vi "Actor Core.vi"(8 "error in":errorcluster, 11 "Camera in":refnum<class "Camera.lvclass">) -> (0 "error out":errorcluster, 3 "Actor out":refnum<class "Actor.lvclass">)   [LabVIEW 2021, in "Camera.lvlib" / "Camera.lvclass"]
doc: "(<B>Filename</B>: Actor Framework.lvlib:Actor.lvclass:Actor Core.vi)\n\nReceives messages to the actor, reacts to them, and initiates any error handling that may shut the actor down.\n\nDescendant classes may override this VI to append parallel tasks for the actor to complete while it handles messages. Overrides use the Call Parent Method node."
uses:
  Camera.lvclass
  C:/Program Files (x86)/National Instruments/LabVIEW 2021/vi.lib/ActorFramework/Actor/Actor.lvclass
  <vilib>/ActorFramework/Actor/Actor.lvclass
  Cam task parameters.ctl
  Display Mode.ctl
  <vilib>/vision/Image Controls.llb/IMAQ Image.ctl
  Utilities/RWC_Actions.ctl
  Camera.lvclass/Camera.ctl
  <vilib>/ActorFramework/Actor/Actor.lvclass/Actor.ctl
  <vilib>/ActorFramework/Message Enqueuer/Message Enqueuer.lvclass/Message Enqueuer.ctl
  Main_Control/Main_Control/notifications.ctl
  Main_Control/Main_Control Messages/UI notifier Msg/UI notifier Msg.lvclass/UI notifier Msg.ctl
  Camera Messages/Cam save image Msg/Cam save image Msg.lvclass/Cam save image Msg.ctl
  <vilib>/ActorFramework/Message Enqueuer/Init from Existing Queue.vi
  <vilib>/ActorFramework/Message Enqueuer/Enqueue.vi
  Camera Messages/Cam change inner param Msg/Cam change inner param Msg.lvclass
  C:/Program Files (x86)/National Instruments/LabVIEW 2021/vi.lib/ActorFramework/Message/Message.lvclass
  Camera Messages/Cam stop task Msg/Cam stop task Msg.lvclass
  Main_Control/Main_Control Messages/UI notifier Msg/UI notifier Msg.lvclass
  Camera Messages/Cam save image Msg/Cam save image Msg.lvclass
  <vilib>/ActorFramework/Message Priority Queue/Priority Enqueue.vi
  <vilib>/ActorFramework/Message Enqueuer/Message Enqueuer.lvclass
  Main_Control/Main_Control/Main_Control.lvclass
panel:
  out "Waveform Graph":dbl[](graph)
  in  "stop":bool
  in  "Change inner param":bool
  in  "Frame Array":T1[](array[typedef])
  in  "Max":u16(slide) scale=0.0..65535.0
  in  "Min":u16(slide) scale=0.0..65535.0
  in  "phase display":i32
  in  "phase#":i32=1
  in  "Display Index":u32(slide) scale=0.0..10.0
  in  "Display Mode":T2
  out "Image":T1(plugin-control)
  in  "Cam task parameters":T3
  out "Current Frame":i32
  out "Exposure Index":i32
  in  "Auto Saving?":bool
  in  "Is Running?":bool
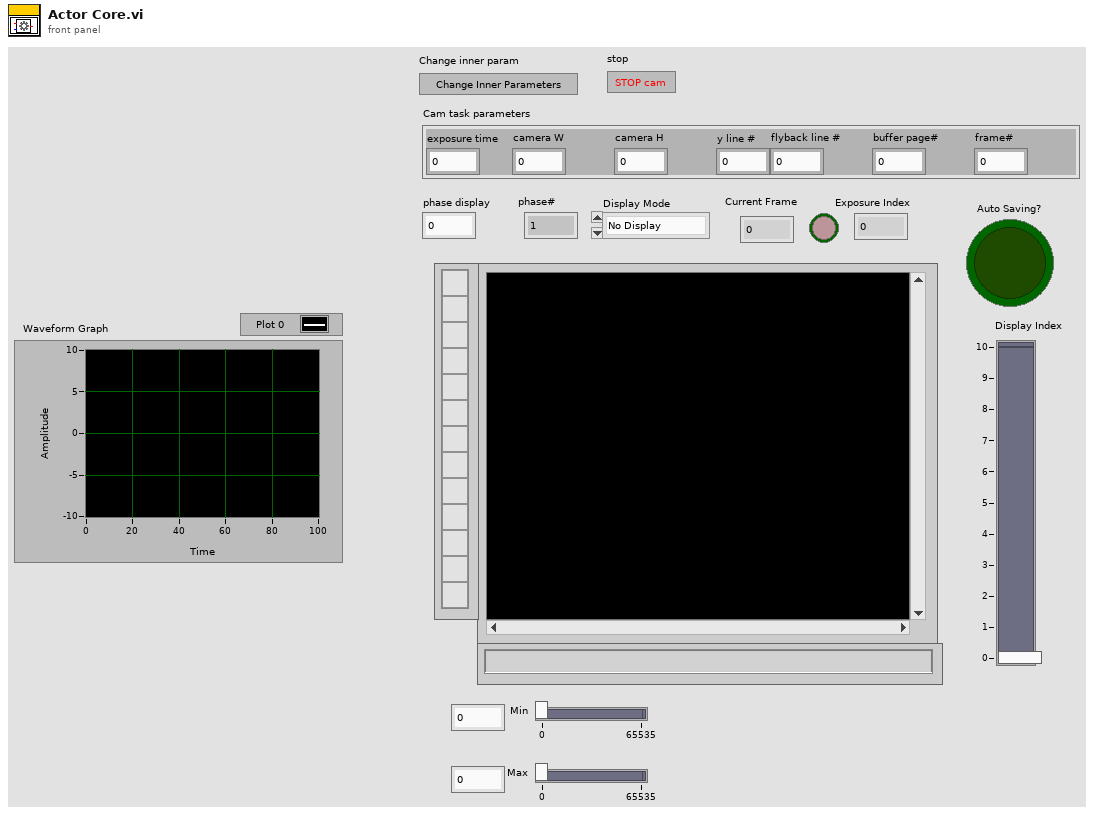
[diagram p1: front panel]
types:
  T1 = typedef "IMAQ Image.ctl" = refnum<image>
  T2 = typedef "Camera.lvlib/Camera.lvclass/Display Mode.ctl" = enum16{"No Display", "Confocal", "Raw Image", "Single Phase", "Line Sum"}
  T3 = typedef "Camera.lvlib/Camera.lvclass/Cam task parameters.ctl" = cluster{"exposure time":dbl, "camera W":dbl, "camera H":dbl, "y line #":dbl, "flyback line #":dbl, "buffer page#":dbl, "frame#":dbl}
  T4 = typedef "RWC_Actions.ctl" = enum16{"Read", "Write", "Read and Create"}
  T5 = typedef "Image Type" = u32
  T6 = typedef "Main_Control.lvlib/Main_Control.lvclass/notifications.ctl" = enum16{"cam 1 frame skkipped", "cam finish", "cam started", "cam stopped", "cam updated", "ni started", "ni stopped", "ni updated"}
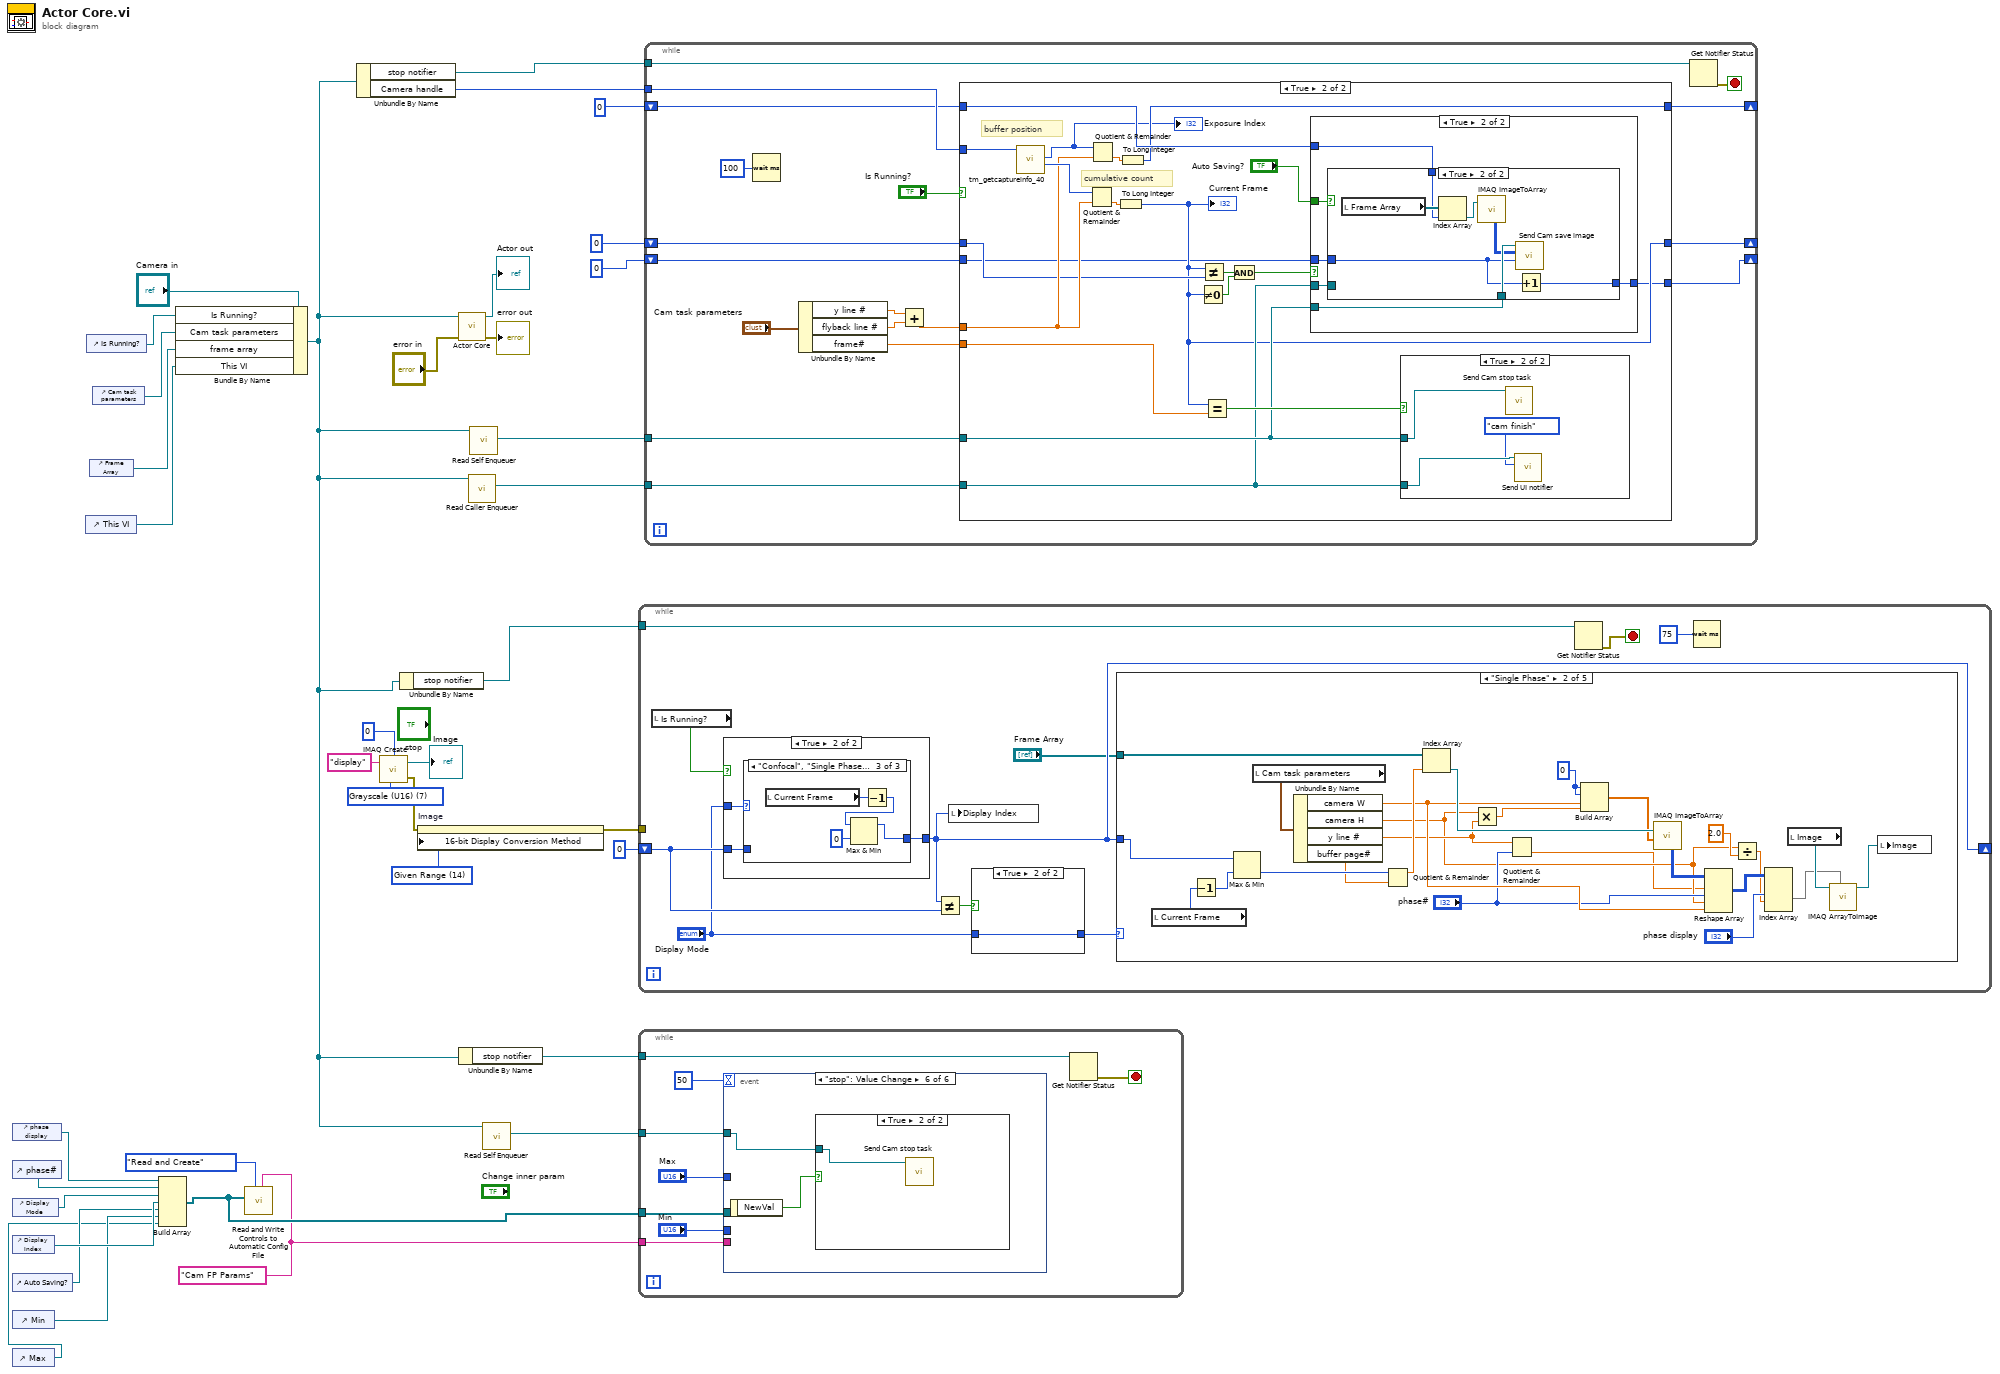
[diagram p0: block diagram]
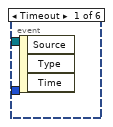
[diagram p2: hidden frame]
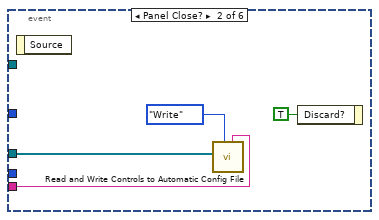
[diagram p3: hidden frame]
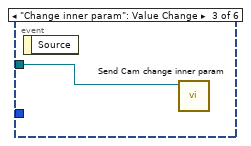
[diagram p4: hidden frame]
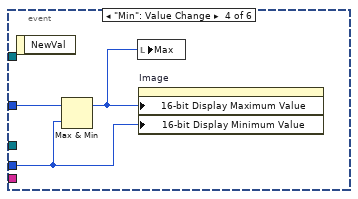
[diagram p5: hidden frame]
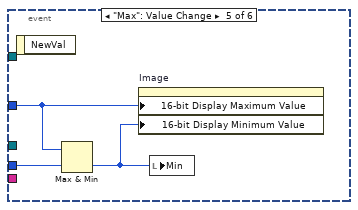
[diagram p6: hidden frame]
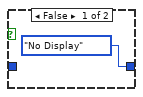
[diagram p8: hidden frame]
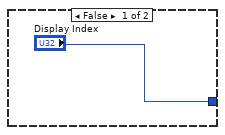
[diagram p9: hidden frame]
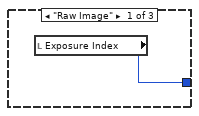
[diagram p10: hidden frame]
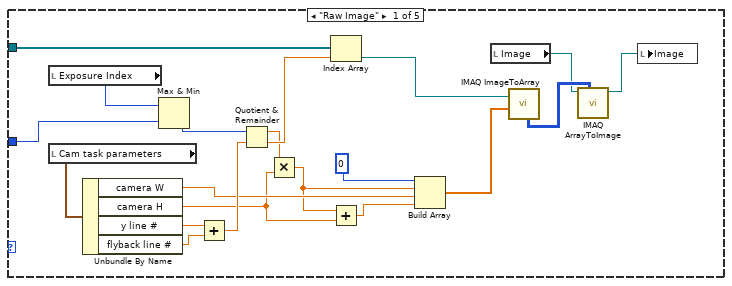
[diagram p12: hidden frame]
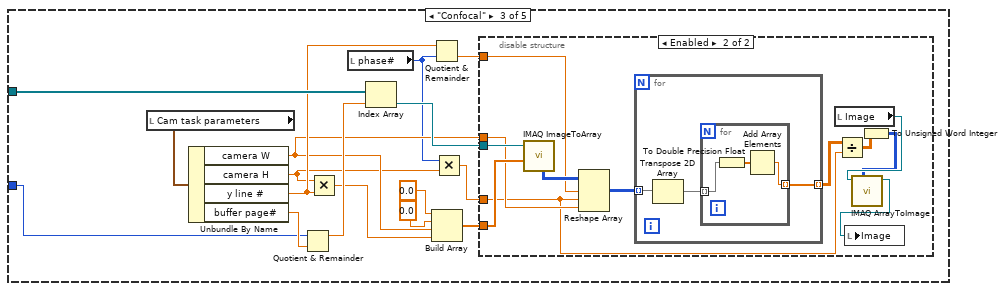
[diagram p13: hidden frame]
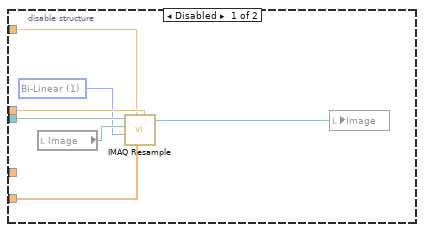
[diagram p14: hidden frame]
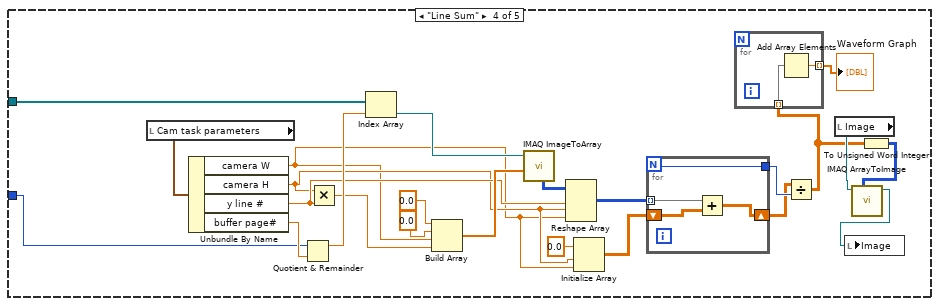
[diagram p15: hidden frame]
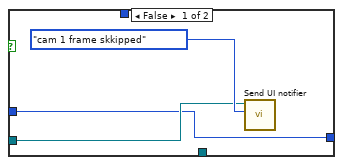
[diagram p20: hidden frame]
diagram:
  w2 = u32 14 items=["Default"=10, "Most Significant Bits"=11, "Full Dynamic"=12, "Downshift"=13, "Given Range"=14, "90% Dynamic"=15, "Given Percent Range"=16] ("16-bit Display Mapping:Conversion Method")
  w5 = "Cam FP Params" ("section (optional)")
  w23 = T5 7 items=["Grayscale (U8)", "Grayscale (I16)", "Grayscale (SGL)", "Complex (CSG)", "RGB (U32)", "HSL (U32)", "RGB (U64)", "Grayscale (U16)"] ("Image Type")
  n1 = control-ref of="phase display"() -> (w14:refnum<vi>)
  n2 = control-ref of="phase#"() -> (w13:refnum<vi>)
  n3 = control-ref of="Display Mode"() -> (w12:refnum<vi>)
  n4 = control-ref of="Display Index"() -> (w11:refnum<vi>)
  n5 = control-ref of="Auto Saving?"() -> (w10:refnum<vi>)
  n6 = control-ref of="Min"() -> (w9:refnum<vi>)
  n7 = control-ref of="Max"() -> (w8:refnum<vi>)
  n8 = control-ref of="This VI"() -> (w18:refnum<vi>)
  n9 = control-ref of="Is Running?"() -> (w34:refnum<vi>)
  n10 = control-ref of="Frame Array"() -> (w20:refnum<vi>)
  n11 = control-ref of="Cam task parameters"() -> (w27:refnum<vi>)
  n12 = Build Array(w14, w13, w12, w11, w10, w9, w8) -> (w6:refnum<vi>[])
  n13 = Bundle By Name(cluster="Camera in", "Is Running?"=w34, "Cam task parameters"=w27, "frame array"=w20, "This VI"=w18) -> (w16:refnum<class "Camera.lvclass">)
  n14 = call "Read and Write Controls to Automatic Config File.vi"("file name"=w5, "Action"=RWC_Actions."Read and Create", "Control References"=w6) -> ()  [unwired: 8 in, 1 out]
  n15 = Unbundle By Name(w16) -> ("stop notifier"=w32:refnum<notifier>, "Camera handle"=w31:u32)
  n16 = call "IMAQ Create"("Border Size"=0, "Image Name"="display", "Image Type"=w23) -> ("New Image"=→"Image":T1, "error out"=w4:errorcluster)  [unwired: 2 in]
  n17 = Unbundle By Name(w16) -> ("stop notifier"=w26:refnum<notifier>)
  n18 = property on="Image" class="ImageControl"(error in=w4, "16-bit Display Conversion Method"=w2) -> (error out=w3:errorcluster)  [unwired: 1 in, 1 out]
  n19 = call-parent "Actor Core.vi"("error in"="error in", "Actor in"=w16) -> ("error out"=→"error out":errorcluster, "Actor out"=→"Actor out":refnum<class "Actor.lvclass">)  [unwired: 8 in]
  n20 = Unbundle By Name(w16) -> ("stop notifier"=w19:refnum<notifier>)
  n21 = call <vilib>:"Read Caller Enqueuer.vi"("Actor"=w16) -> ("Caller Enqueuer"=w15:refnum<class "Message Enqueuer.lvclass">)  [unwired: 10 in]
  n22 = call <vilib>:"Read Self Enqueuer.vi"("Actor"=w16) -> ("Self Enqueuer"=w29:refnum<class "Message Enqueuer.lvclass">)  [unwired: 10 in]
  n23 = call <vilib>:"Read Self Enqueuer.vi"("Actor"=w16) -> ("Self Enqueuer"=w17:refnum<class "Message Enqueuer.lvclass">)  [unwired: 10 in]
  n24 = while {
    tunnel: w26 -> [w46]
    tunnel: w3 -> [_]
    shift-right: [w39] -> _
    shift-left: u32 0 ("Display Index") -> [w43]
    stop <- w47 stop-if-true
    n25 = local read "Is Running?"() -> (w44:bool)
    n26 = case shown="True" w44 {
      tunnel: ["Display Index" w53] -> w39
      tunnel: "Display Mode" -> [_ w52]
      tunnel: w43 -> [_ w51]
      frame False {
      }
      frame True {
        n27 = case shown="\"Confocal\", \"Single Phase\", \"Line Sum\"" w52 {
          tunnel: [w54 w55 w56] -> w53
          tunnel: w51 -> [_ w55 _]
          frame "Raw Image" {
            n28 = local read "Exposure Index"() -> (w54:i32)
          }
          frame "No Display" {
          }
          frame "Confocal", "Single Phase", "Line Sum" {
            n29 = local read "Current Frame"() -> (w59:i32)
            n30 = Decrement(x=w59) -> (x-1=w58:i32)
            n31 = Max & Min(x=w58, y=0) -> (max(x,y)=w56:i32)  [unwired: 1 out]
          }
        }
      }
    }
    n32 = Not Equal?(x=w39, y=w43) -> (x != y?=w42:bool)
    n33 = local write "Display Index"(w39) -> ()
    n34 = case shown="True" w42 {
      tunnel: "Display Mode" -> [_ w49]
      tunnel: [Display_Mode."No Display" ("Display Mode") w49] -> w40
      frame False {
      }
      frame True {
      }
    }
    n35 = case shown="\"Single Phase\"" w40 {
      tunnel: "Frame Array" -> [w75 w104 w120 w169 _]
      tunnel: w39 -> [w68 w101 w111 w162 _]
      frame "Raw Image" {
        n36 = local read "Exposure Index"() -> (w69:i32)
        n37 = local read "Cam task parameters"() -> (w79:T3)
        n38 = Unbundle By Name(w79) -> ("camera W"=w72:dbl, "camera H"=w65:dbl, "y line #"=w78:dbl, "flyback line #"=w77:dbl)
        n39 = Max & Min(x=w69, y=w68) -> (min(x,y)=w70:u32)  [unwired: 1 out]
        n40 = Add(x=w78, y=w77) -> (x+y=w76:dbl)
        n41 = Quotient & Remainder(x=w70, y=w76) -> (x-y*floor(x/y)=w66:dbl, floor(x/y)=w74:dbl)
        n42 = Multiply(x=w66, y=w65) -> (x*y=w67:dbl)
        n43 = Index Array(array=w75, index=w74) -> (element=w64:T1)
        n44 = Add(x=w67, y=w65) -> (x+y=w71:dbl)
        n45 = Build Array(0, w67, w72, w71) -> (w63:dbl[])
        n46 = local read "Image"() -> (w61:T1)
        n47 = call "IMAQ ImageToArray"("Optional Rectangle"=w63, "Image"=w64) -> ("Image Pixels (U16)"=w62:u16[][])  [unwired: 2 in, 4 out]
        n48 = call "IMAQ ArrayToImage"("Image Pixels (U16)"=w62, "Image"=w61) -> ("Image Out"=w60:T1)  [unwired: 8 in, 1 out]
        n49 = local write "Image"(w60) -> ()
      }
      frame "Single Phase" {
        w90 = 0
        n50 = local read "Current Frame"() -> (w102:i32)
        n51 = Decrement(x=w102) -> (x-1=w100:i32)
        n52 = Max & Min(x=w101, y=w100) -> (min(x,y)=w103:u32)  [unwired: 1 out]
        n53 = local read "Cam task parameters"() -> (w99:T3)
        n54 = Unbundle By Name(w99) -> ("camera W"=w89:dbl, "camera H"=w82:dbl, "y line #"=w88:dbl, "buffer page#"=w98:dbl)
        n55 = Quotient & Remainder(x=w103, y=w98) -> (x-y*floor(x/y)=w97:dbl)  [unwired: 1 out]
        n56 = Index Array(array=w104, index=w97) -> (element=w93:T1)
        n57 = Multiply(x=w82, y=w88) -> (x*y=w96:dbl)
        n58 = Quotient & Remainder(x=w88, y="phase#") -> (floor(x/y)=w81:dbl)  [unwired: 1 out]
        n59 = Build Array(w90, w90, w89, w96) -> (w92:dbl[])
        n60 = call "IMAQ ImageToArray"("Optional Rectangle"=w92, "Image"=w93) -> ("Image Pixels (U16)"=w91:u16[][])  [unwired: 2 in, 4 out]
        n61 = Reshape Array(w91, w81, "phase#", w82, w89) -> (w86:u16[][][][])
        n62 = Divide(x=w82, y=2.0) -> (x/y=w80:dbl)
        n63 = Index Array(array=w86, index (dim 1)="phase display", index (dim 2)=w80) -> (element=w83:u16[][])  [unwired: 2 in]
        n64 = local read "Image"() -> (w95:T1)
        n65 = call "IMAQ ArrayToImage"("Image Pixels (U16)"=w83, "Image"=w95) -> ("Image Out"=w94:T1)  [unwired: 8 in, 1 out]
        n66 = local write "Image"(w94) -> ()
      }
      frame "Confocal" {
        n67 = local read "Cam task parameters"() -> (w119:T3)
        n68 = Unbundle By Name(w119) -> ("camera W"=w112:dbl, "camera H"=w106:dbl, "y line #"=w113:dbl, "buffer page#"=w118:dbl)
        n69 = Quotient & Remainder(x=w111, y=w118) -> (x-y*floor(x/y)=w117:dbl)  [unwired: 1 out]
        n70 = Multiply(x=w106, y=w113) -> (x*y=w114:dbl)
        n71 = local read "phase#"() -> (w107:i32)
        n72 = Index Array(array=w120, index=w117) -> (element=w115:T1)
        n73 = Quotient & Remainder(x=w113, y=w107) -> (floor(x/y)=w110:dbl)  [unwired: 1 out]
        n74 = Build Array(0.0 ("element"), 0.0 ("element"), w112, w114) -> (w109:dbl[])
        n75 = Multiply(x=w107, y=w106) -> (x*y=w105:dbl)
        n76 = disable-structure shown="Enabled" {
          disable-tunnel: w115 -> [w127 w139]
          disable-tunnel: w112 -> [w126 w135]
          disable-tunnel: w110 -> [w125 w136]
          disable-tunnel: w109 -> [w124 w138]
          disable-tunnel: w105 -> [_ w128]
          frame Disabled {
            w121 = u32 1 items=["Zero Order", "Bi-Linear", "Quadratic", "Cubic Spline"] ("Interpolation Type")
            n77 = local read "Image"() -> (w123:T1)
            n78 = call "IMAQ Resample"("X Resolution"=w126, "Optional Rectangle"=w124, "Y Resolution"=w125, "Interpolation Type"=w121, "Image Dst"=w123, "Image Src"=w127) -> ("Image Dst Out"=w122:T1)  [unwired: 4 in, 1 out]
            n79 = local write "Image"(w122) -> ()
          }
          frame Enabled {
            n80 = call "IMAQ ImageToArray"("Optional Rectangle"=w138, "Image"=w139) -> ("Image Pixels (U16)"=w137:u16[][])  [unwired: 2 in, 4 out]
            n81 = Reshape Array(w137, w136, w128, w135) -> (w134:u16[][][])
            n82 = for {
              tunnel: w134 -> [w142] mode=indexing
              tunnel: [w140] -> w131 mode=indexing
              n83 = Transpose 2D Array(2D array=w142) -> (transposed array=w141:u16[][])
              n84 = for {
                tunnel: w141 -> [w144] mode=indexing
                tunnel: [w145] -> w140 mode=indexing
                n85 = To Double Precision Float(number=w144) -> (double precision float=w143:dbl[])
                n86 = Add Array Elements(numeric array=w143) -> (sum=w145:dbl)
              }
            }
            n87 = local read "Image"() -> (w133:T1)
            n88 = Divide(x=w131, y=w128) -> (x/y=w130:dbl[][])
            n89 = To Unsigned Word Integer(number=w130) -> (unsigned 16bit integer=w129:u16[][])
            n90 = call "IMAQ ArrayToImage"("Image Pixels (U16)"=w129, "Image"=w133) -> ("Image Out"=w132:T1)  [unwired: 8 in, 1 out]
            n91 = local write "Image"(w132) -> ()
          }
        }
      }
      frame "Line Sum" {
        n92 = local read "Cam task parameters"() -> (w168:T3)
        n93 = Unbundle By Name(w168) -> ("camera W"=w151:dbl, "camera H"=w152:dbl, "y line #"=w154:dbl, "buffer page#"=w167:dbl)
        n94 = Quotient & Remainder(x=w162, y=w167) -> (x-y*floor(x/y)=w166:dbl)  [unwired: 1 out]
        n95 = Multiply(x=w152, y=w154) -> (x*y=w163:dbl)
        n96 = Index Array(array=w169, index=w166) -> (element=w164:T1)
        n97 = Build Array(0.0 ("element"), 0.0 ("element"), w151, w163) -> (w161:dbl[])
        n98 = call "IMAQ ImageToArray"("Optional Rectangle"=w161, "Image"=w164) -> ("Image Pixels (U16)"=w159:u16[][])  [unwired: 2 in, 4 out]
        n99 = Reshape Array(w159, w154, w152, w151) -> (w158:u16[][][])
        n100 = Initialize Array(0.0 ("element"), w152, w151) -> (w150:dbl[][])
        n101 = for {
          N -> [w172]
          tunnel: w158 -> [w174] mode=indexing
          shift-right: [w175] -> w148
          shift-left: w150 -> [w173]
          tunnel: [w172] -> w149
          n102 = Add(x=w174, y=w173) -> (x+y=w175:dbl[][])
        }
        n103 = Divide(x=w148, y=w149) -> (x/y=w147:dbl[][])
        n104 = for {
          tunnel: w147 -> [w171] mode=indexing
          tunnel: [w170] -> w146 mode=indexing
          n105 = Add Array Elements(numeric array=w171) -> (sum=w170:dbl)
        }
        "Waveform Graph" <- w146
        n106 = local read "Image"() -> (w157:T1)
        n107 = To Unsigned Word Integer(number=w147) -> (unsigned 16bit integer=w155:u16[][])
        n108 = call "IMAQ ArrayToImage"("Image Pixels (U16)"=w155, "Image"=w157) -> ("Image Out"=w156:T1)  [unwired: 8 in, 1 out]
        n109 = local write "Image"(w156) -> ()
      }
      frame "No Display", Default {
      }
    }
    n110 = Get Notifier Status(notifier=w46) -> (error out=w47:errorcluster)  [unwired: 1 in, 4 out]
    n111 = Wait (ms)(milliseconds to wait=u32 75) -> ()  [unwired: 1 out]
  }
  n112 = while {
    tunnel: w19 -> [w183]
    tunnel: w17 -> [w178]
    tunnel: w6 -> [w177]
    tunnel: w5 -> [w176]
    stop <- w182 stop-if-true
    n113 = event shown="[5] \"stop\": Value Change" {
      selector: _ -> [_ _ _ _ _ _]
      dyn-events: _ -> [_ _ _ _ _ _]
      timeout: 50 -> [_ _ _ _ _ _]
      tunnel: "Min" -> [_ _ _ w191 w194 _]
      tunnel: "Max" -> [_ _ _ w189 w193 _]
      tunnel: w178 -> [_ _ w188 _ _ w195]
      tunnel: w177 -> [_ w186 _ _ _ _]
      tunnel: w176 -> [_ w184 _ _ _ _]
      event Timeout {
        n114 = event-data() -> ()  [unwired: 1 in, 3 out]
      }
      event Panel Close? {
        n115 = event-data() -> ()  [unwired: 1 in, 1 out]
        n116 = call "Read and Write Controls to Automatic Config File.vi"("file name"=w184, "Action"=RWC_Actions."Write", "Control References"=w186) -> ()  [unwired: 8 in, 1 out]
        n117 = event-data("Discard?"=TRUE) -> ()  [unwired: 1 in, 1 out]
      }
      event "Change inner param": Value Change {
        n118 = event-data() -> ()  [unwired: 1 in, 1 out]
        n119 = call "Send Cam change inner param.vi"("Message Enqueuer"=w188) -> ()  [unwired: 9 in, 2 out]
      }
      event "Min": Value Change {
        n120 = event-data() -> ()  [unwired: 1 in, 1 out]
        n121 = Max & Min(x=w189, y=w191) -> (max(x,y)=w190:u16)  [unwired: 1 out]
        n122 = local write "Max"(w190) -> ()
        n123 = property on="Image" class="ImageControl"("16-bit Display Maximum Value"=w190, "16-bit Display Minimum Value"=w191) -> ()  [unwired: 2 in, 2 out]
      }
      event "Max": Value Change {
        n124 = event-data() -> ()  [unwired: 1 in, 1 out]
        n125 = Max & Min(x=w193, y=w194) -> (min(x,y)=w192:u16)  [unwired: 1 out]
        n126 = property on="Image" class="ImageControl"("16-bit Display Maximum Value"=w193, "16-bit Display Minimum Value"=w192) -> ()  [unwired: 2 in, 2 out]
        n127 = local write "Min"(w192) -> ()
      }
      event "stop": Value Change {
        n128 = event-data() -> ("NewVal"=w196:bool)  [unwired: 1 in]
        n129 = case shown="True" w196 {
          tunnel: w195 -> [_ w197]
          frame False {
          }
          frame True {
            n130 = call "Send Cam stop task.vi"("Message Enqueuer"=w197) -> ()  [unwired: 9 in, 2 out]
          }
        }
      }
    }
    n131 = Get Notifier Status(notifier=w183) -> (error out=w182:errorcluster)  [unwired: 1 in, 4 out]
  }
  n132 = while {
    tunnel: w32 -> [w215]
    tunnel: w31 -> [w214]
    shift-right: [w211] -> _
    shift-left: 0 ("Frame Count") -> [w212]
    shift-right: [w209] -> _
    shift-left: 0 ("Frame Count") -> [w210]
    tunnel: w29 -> [w208]
    tunnel: w15 -> [w201]
    shift-right: [w198] -> _
    shift-left: 0 ("Frame Count") -> [w199]
    stop <- w213 stop-if-true
    n133 = Wait (ms)(milliseconds to wait=u32 100) -> ()  [unwired: 1 out]
    n134 = Unbundle By Name("Cam task parameters") -> ("y line #"=w204:dbl, "flyback line #"=w205:dbl, "frame#"=w202:dbl)
    n135 = Add(x=w204, y=w205) -> (x+y=w203:dbl)
    n136 = case shown="True" "Is Running?" {
      tunnel: w214 -> [_ w225]
      tunnel: w203 -> [_ w237]
      tunnel: w212 -> [w218 w235]
      tunnel: [w218 w221] -> w211
      tunnel: w210 -> [w217 w233]
      tunnel: [w217 w232] -> w209
      tunnel: w202 -> [_ w231]
      tunnel: w208 -> [_ w228]
      tunnel: w201 -> [_ w226]
      tunnel: w199 -> [w216 w220]
      tunnel: [w216 w219] -> w198
      frame False {
      }
      frame True {
        # "cumulative count"
        # "buffer position"
        n137 = call <userlib>:"tm_getcaptureinfo_40.vi"("Handle in"=w225) -> ("Frame Count"=w238:i32, "Frame Index"=w229:i32)  [unwired: 7 in, 2 out]
        "Exposure Index" <- w229
        n138 = Quotient & Remainder(x=w238, y=w237) -> (floor(x/y)=w236:dbl)  [unwired: 1 out]
        n139 = Quotient & Remainder(x=w229, y=w237) -> (floor(x/y)=w234:dbl)  [unwired: 1 out]
        n140 = To Long Integer(number=w236) -> (32bit integer=w221:i32)
        "Current Frame" <- w221
        n141 = To Long Integer(number=w234) -> (32bit integer=w232:i32)
        n142 = Not Equal To 0?(x=w221) -> (x != 0?=w222:bool)
        n143 = Not Equal?(x=w221, y=w235) -> (x != y?=w224:bool)
        n144 = Equal?(x=w221, y=w231) -> (x = y?=w230:bool)
        n145 = And(x=w224, y=w222) -> (x .and. y?=w223:bool)
        n146 = case shown="True" w223 {
          tunnel: w233 -> [_ w248]
          tunnel: w228 -> [_ w247]
          tunnel: "Auto Saving?" -> [_ w246]
          tunnel: w226 -> [_ w245]
          tunnel: w220 -> [w242 w244]
          tunnel: [w242 w243] -> w219
          frame False {
          }
          frame True {
            n147 = case shown="True" w246 {
              tunnel: w248 -> [_ w254]
              tunnel: w247 -> [_ w258]
              tunnel: w245 -> [w250 _]
              tunnel: w244 -> [w249 w257]
              tunnel: [w249 w256] -> w243
              frame False {
                n148 = call "Send UI notifier.vi"("Object&State"=notifications."cam 1 frame skkipped", "Message Enqueuer"=w250) -> ()  [unwired: 8 in, 2 out]
              }
              frame True {
                n149 = local read "Frame Array"() -> (w255:T1[])
                n150 = Index Array(array=w255, index=w254) -> (element=w253:T1)
                n151 = call "IMAQ ImageToArray"("Image"=w253) -> ("Image Pixels (U16)"=w252:u16[][])  [unwired: 3 in, 4 out]
                n152 = call "Send Cam save image.vi"("file index"=w257, "page"=w252, "Message Enqueuer"=w258) -> ()  [unwired: 7 in, 2 out]
                n153 = Increment(x=w257) -> (x+1=w256:i32)
              }
            }
          }
        }
        n154 = case shown="True" w230 {
          tunnel: w228 -> [_ w239]
          tunnel: w226 -> [_ w241]
          frame False {
          }
          frame True {
            n155 = call "Send Cam stop task.vi"("Message Enqueuer"=w239) -> ()  [unwired: 9 in, 2 out]
            n156 = call "Send UI notifier.vi"("Object&State"=notifications."cam finish", "Message Enqueuer"=w241) -> ()  [unwired: 8 in, 2 out]
          }
        }
      }
    }
    n157 = Get Notifier Status(notifier=w215) -> (error out=w213:errorcluster)  [unwired: 1 in, 4 out]
  }
